vi "Import Frames RTM.vi"(8 "error in":errorcluster, 11 "Node Ptr":T1 format="%.0x") -> (0 "error out":errorcluster)   [LabVIEW 2020, in "Ballard MIL-STD-1553 System Explorer.lvlib" / "Implementation.lvlib"]
doc: "This VI runs when the Import Frames run-time menu is chosen. It allows the user to import frames from the database associated with the port that will contain these frames."
uses:
  Implementation.lvlib
  <vilib>/NI VeriStand/Custom Device API/Custom Device Item Ref.ctl
  <vilib>/NI VeriStand/Custom Device API/Custom Device Channel.ctl
  <vilib>/NI VeriStand/Custom Device API/Custom Device Channel Type.ctl
  Scripting/Constants.vi
  <vilib>/NI VeriStand/Custom Device Tools/Custom Device Utility Library/Custom Device Utility Library.lvlib
  <vilib>/NI VeriStand/Custom Device API/Custom Device API.lvlib
  Scripting/Ballard MIL-STD-1553 Scripting.lvlib
panel:
  in  "Select Frames":i32[](listbox)
  out "Database":string
  in  "Help":bool
  in  "Cancel":bool
  in  "OK":bool
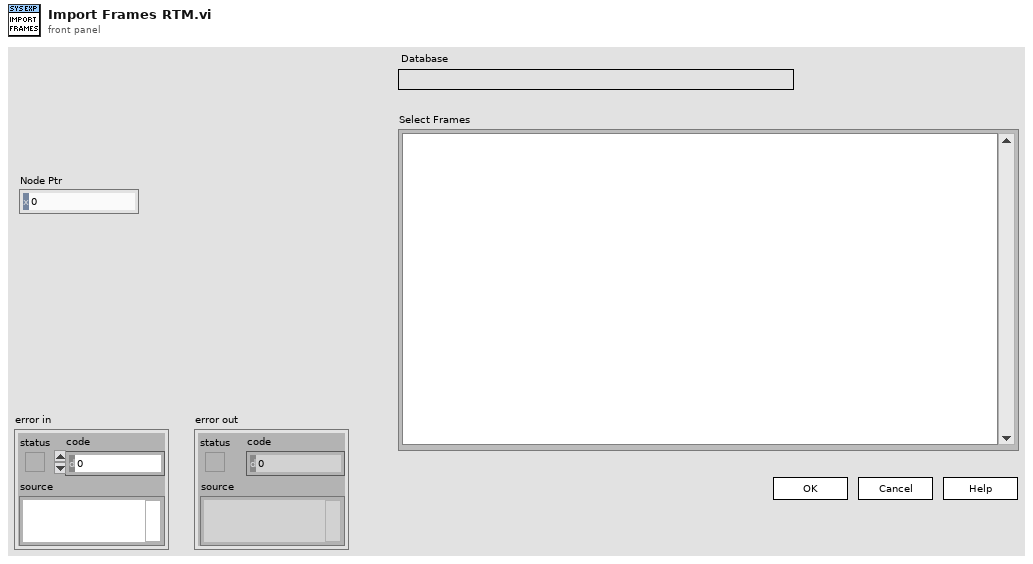
[diagram p1: front panel]
types:
  T1 = typedef "Custom Device API.lvlib/Custom Device Item Ref.ctl" = u64
  T2 = typedef "Custom Device API.lvlib/Custom Device Channel.ctl" = cluster{"Type":T3, "Units":string, "Default Value":dbl, "Faultable":bool, "Scalable":bool}
  T3 = typedef "Custom Device API.lvlib/Custom Device Channel Type.ctl" = enum16{"Input", "Output"}
  T4 = typedef "Ballard MIL-STD-1553 System Explorer.lvlib/Implementation.lvlib/Database.ctl" = cluster{"Baud Rate":u64, "Frames":cluster{"Name":string, "ID":i32}[]}
  T5 = cluster{"Channel":T2, "Node Ptr":T1, "Frames":cluster{"Name":string, "ID":i32}[]}
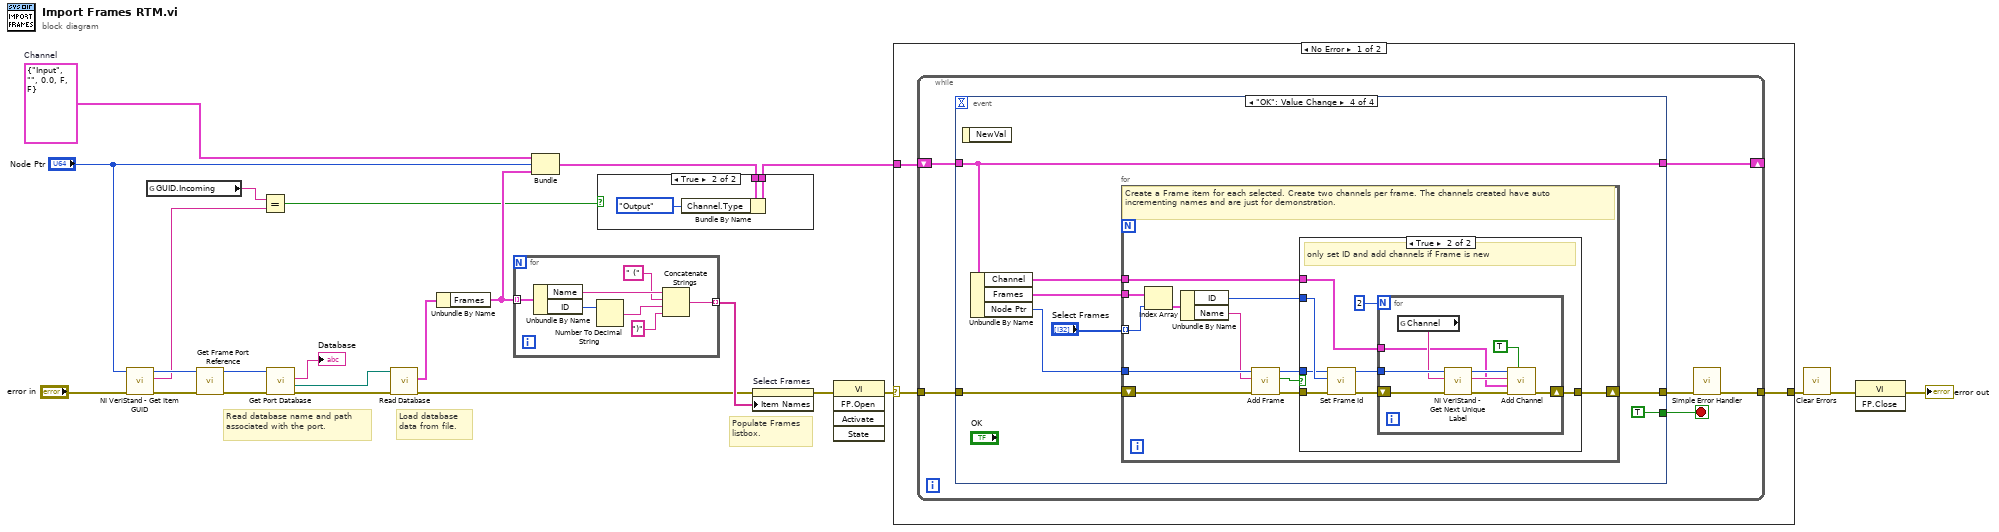
[diagram p0: block diagram]
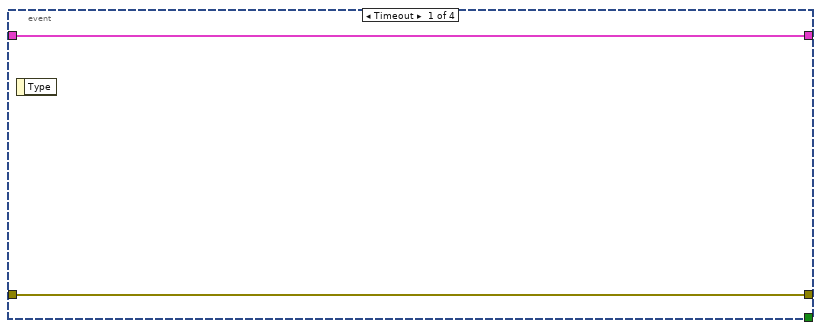
[diagram p2: hidden frame]
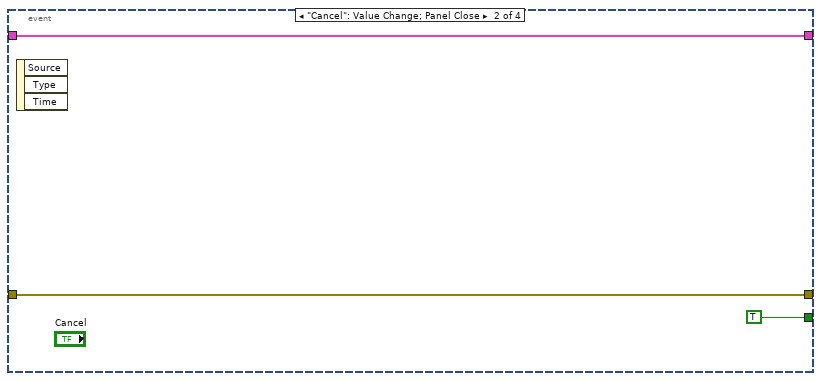
[diagram p3: hidden frame]
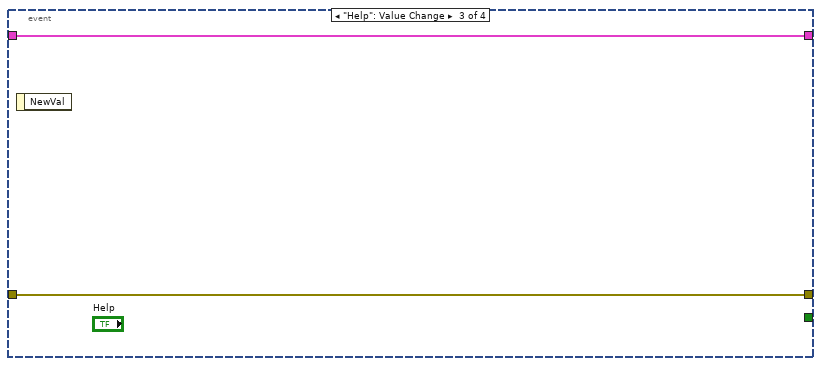
[diagram p4: hidden frame]
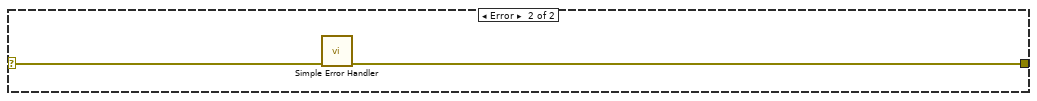
[diagram p6: hidden frame]
diagram:
  w12 = T2 {"Type"=enum."Input", "Units"="", "Default Value"=0.0, "Faultable"=FALSE, "Scalable"=FALSE}  # Channel
  # "Populate Frames listbox."
  # "Load database data from file."
  # "Read database name and path associated with the port."
  n1 = call <vilib>:"NI VeriStand - Get Item GUID.vi"("error in (no error)"="error in", "Item Ref in"="Node Ptr") -> ("error out"=w14:errorcluster, "GUID"=w8:string, "Item Ref out"=w13:T1)  [unwired: 7 in]
  n2 = global read "Constants.vi" "GUID.Incoming"() -> (w9:string)
  n3 = call "Get Frame Port Reference.vi"("error in"=w14, "Frame Ref"=w13) -> ("error out"=w6:errorcluster, "Port Ref"=w5:T1)  [unwired: 8 in]
  n4 = Equal?(x=w9, y=w8) -> (x = y?=w7:bool)
  n5 = call "Get Port Database.vi"("error in"=w6, "Port Ref"=w5) -> ("error out"=w3:errorcluster, "Database Path"=w2:path, "Database Name"=→"Database":string)  [unwired: 5 in, 2 out]
  n6 = call "Read Database.vi"("error in"=w3, "Path"=w2) -> ("error out"=w18:errorcluster, "Database"=w21:T4)  [unwired: 8 in]
  n7 = Unbundle By Name(w21) -> ("Frames"=w19:cluster{"Name":string, "ID":i32}[])
  n8 = for {
    tunnel: w19 -> [w31] mode=indexing
    tunnel: [w25] -> w20 mode=indexing
    n9 = Unbundle By Name(w31) -> ("Name"=w29:string, "ID"=w30:i32)
    n10 = Number To Decimal String(number=w30) -> (decimal integer string=w27:string)  [unwired: 1 in]
    n11 = Concatenate Strings(w29, " (" ("string"), w27, ")" ("string")) -> (w25:string)
  }
  n12 = Bundle("Channel"=w12, "Node Ptr"="Node Ptr", "Frames"=w19) -> (w11:T5)  [unwired: 1 in]
  n13 = case shown="True" w7 {
    tunnel: w11 -> [w32 w34]
    tunnel: [w32 w33] -> w10
    frame False {
    }
    frame True {
      n14 = Bundle By Name(cluster=w34, "Channel.Type"=Custom_Device_Channel_Type."Output") -> (w33:T5)
    }
  }
  n15 = property on="Select Frames" class="LstBox (strict)"(error in=w18, "Item Names"=w20) -> (error out=w16:errorcluster)  [unwired: 1 in, 1 out]
  n16 = invoke class="VI" method="FP.Open"(error in=w16) -> (error out=w17:errorcluster)  [unwired: 4 in, 4 out]
  n17 = case shown="No Error" w17 {
    selector: w17 -> [w38 w91]
    tunnel: [w37 w90] -> w24
    tunnel: w10 -> [w36 _]
    frame No Error {
      n18 = while {
        tunnel: w38 -> [w44]
        tunnel: [w42] -> w37
        shift-right: [w39] -> _
        shift-left: w36 -> [w40]
        stop <- w41 stop-if-true
        n19 = event shown="[3] \"OK\": Value Change" {
          selector: _ -> [_ _ _ _]
          dyn-events: _ -> [_ _ _ _]
          timeout: _ -> [_ _ _ _]
          tunnel: [w46 w48 w51 w55] -> w43
          tunnel: w44 -> [w46 w48 w51 w58]
          tunnel: [_ TRUE ("Discard?") _ TRUE ("Discard?")] -> w41
          tunnel: w40 -> [w45 w47 w50 w57]
          tunnel: [w45 w47 w50 w57] -> w39
          event Timeout {
            n20 = event-data() -> ()  [unwired: 1 in, 1 out]
          }
          event "Cancel": Value Change; Panel Close {
            n21 = event-data() -> ()  [unwired: 1 in, 3 out]
          }
          event "Help": Value Change {
            n22 = event-data() -> ()  [unwired: 1 in, 1 out]
          }
          event "OK": Value Change {
            n23 = event-data() -> ()  [unwired: 1 in, 1 out]
            n24 = Unbundle By Name(w57) -> ("Channel"=w52:T2, "Frames"=w54:cluster{"Name":string, "ID":i32}[], "Node Ptr"=w56:T1)
            n25 = for {
              tunnel: w56 -> [w70]
              shift-right: [w63] -> w55
              shift-left: w58 -> [w71]
              tunnel: w54 -> [w69]
              tunnel: "Select Frames" -> [w68] mode=indexing
              tunnel: w52 -> [w64]
              # "Create a Frame item for each selected. Create two channels per frame. The channels created have auto incrementing names and are just for demonstration."
              n26 = Index Array(array=w69, index=w68) -> (element=w67:cluster{"Name":string, "ID":i32})
              n27 = Unbundle By Name(w67) -> ("ID"=w65:i32, "Name"=w66:string)
              n28 = call "Add Frame.vi"("error in"=w71, "Name"=w66, "Port Ref"=w70) -> ("error out"=w62:errorcluster, "Newly Created?"=w60:bool, "Frame Ref out"=w61:T1)  [unwired: 6 in]
              n29 = case shown="True" w60 {
                tunnel: w65 -> [_ w80]
                tunnel: w64 -> [_ w76]
                tunnel: [w72 w75] -> w63
                tunnel: w62 -> [w72 w74]
                tunnel: w61 -> [_ w73]
                frame False {
                }
                frame True {
                  # "only set ID and add channels if Frame is new"
                  n30 = call "Set Frame Id.vi"("error in"=w74, "ID"=w80, "Frame Ref"=w73) -> ("error out"=w78:errorcluster, "Frame Ref out"=w77:T1)  [unwired: 7 in]
                  n31 = for {
                    N: 2 -> [_]
                    shift-right: [w88] -> w75
                    shift-left: w78 -> [w89]
                    tunnel: w77 -> [w85]
                    tunnel: w76 -> [w81]
                    n32 = global read "Constants.vi" "Channel"() -> (w84:string)
                    n33 = call <vilib>:"NI VeriStand - Get Next Unique Label.vi"("error in (no error)"=w89, "Label"=w84, "Parent Ref in"=w85) -> ("error out"=w87:errorcluster, "Label out"=w83:string, "Parent Ref dup"=w86:T1)  [unwired: 5 in, 1 out]
                    n34 = call "Add Channel.vi"("Highlight? (F)"=TRUE, "error in"=w87, "Channel"=w81, "Name"=w83, "Frame Ref"=w86) -> ("error out"=w88:errorcluster)  [unwired: 5 in, 1 out]
                  }
                }
              }
            }
          }
        }
        n35 = call <vilib>:"Simple Error Handler.vi"("error in (no error)"=w43) -> ("error out"=w42:errorcluster)  [unwired: 4 in, 4 out]
      }
    }
    frame Error {
      n36 = call <vilib>:"Simple Error Handler.vi"("error in (no error)"=w91) -> ("error out"=w90:errorcluster)  [unwired: 4 in, 4 out]
    }
  }
  n37 = call <vilib>:"Clear Errors.vi"("error in (no error)"=w24) -> ("error out"=w23:errorcluster)  [unwired: 5 in, 1 out]
  n38 = invoke class="VI" method="FP.Close"(error in=w23) -> (error out=→"error out":errorcluster)  [unwired: 2 in, 2 out]
